vi "subTwoAntennaAlamoutiReceiver.vi"(0 "symbols in":cdb[][](array[numeric]) format="%#_6p", 5 "channel estimate":cdb[][][](array[numeric]) format="%#_6p", 11 "error in (no error)":errorcluster) -> (4 "symbols out":cdb[](array[numeric]) format="%#_6p", 15 "error out":errorcluster)   [LabVIEW 2011]
uses:
  <vilib>/Analysis/baseanly.llb/Complex A x B.vi
  <vilib>/Analysis/NI_AALBase.lvlib
panel:
  out "h matrix":cdb[][](array[numeric])
  out "branch SNRs":dbl[][](array[numeric]) format="%#_6p"
  out "combiner SNR":dbl format="%#_6p"
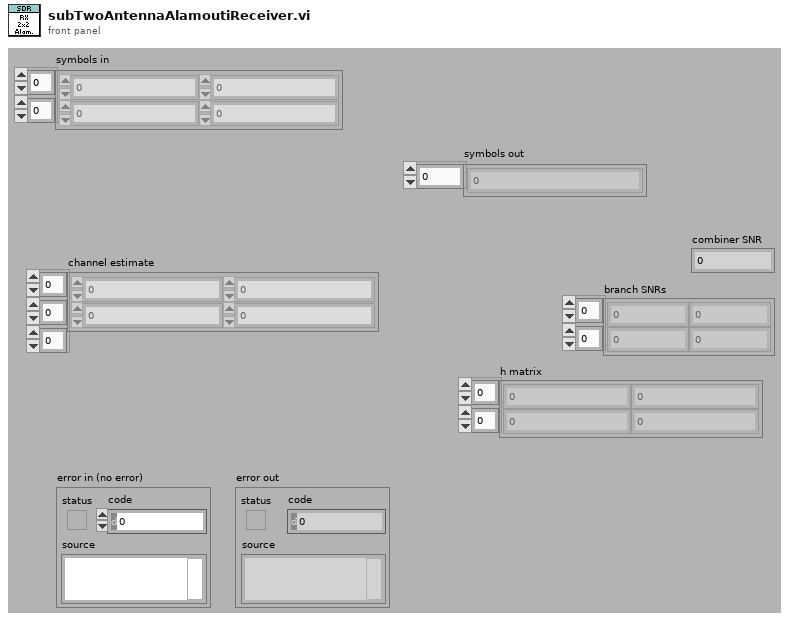
[diagram p1: front panel]
types:
  T1 = typedef "NI_Matrix.lvlib/ComplexMatrix.ctl" = cdb[][]
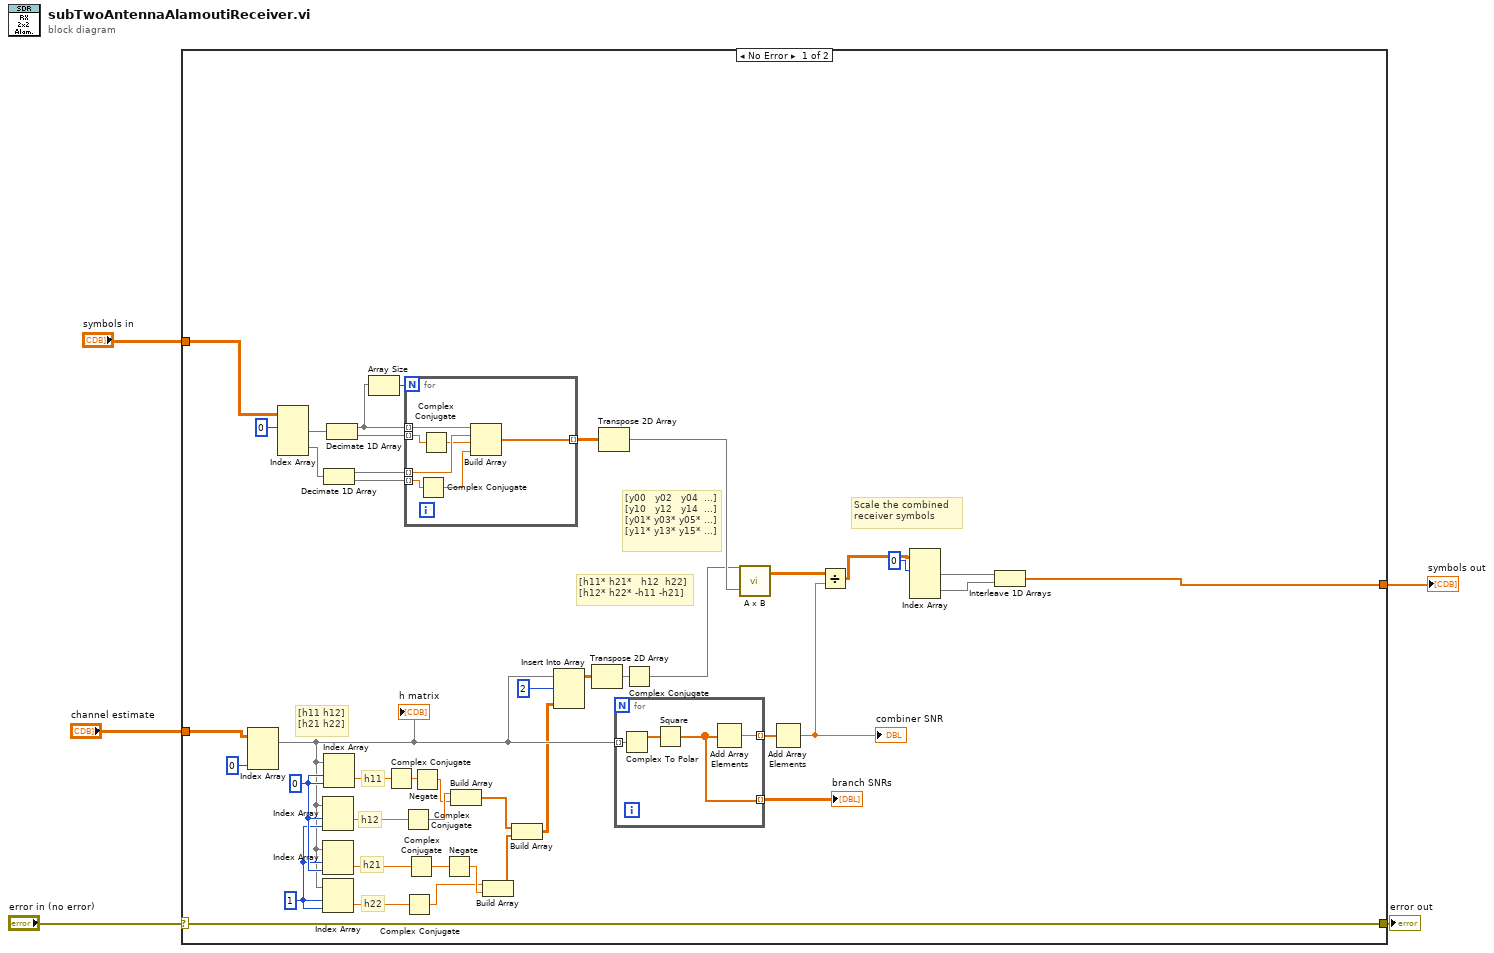
[diagram p0: block diagram]
diagram:
  n1 = case shown="No Error" "error in (no error)" {
    selector: "error in (no error)" -> [w47 w60]
    tunnel: [w47 w60] -> w4
    tunnel: "symbols in" -> [w13 _]
    tunnel: "channel estimate" -> [w12 _]
    tunnel: [w11 _] -> w1
    frame No Error {
      w42 = 1 ("index (row)")
      w43 = 0 ("index (row)")
      # "[h11* h21*   h12  h22]\n[h12* h22* -h11 -h21]"
      # "[y00   y02   y04  ...]\n[y10   y12   y14  ...]\n[y01* y03* y05* ...]\n[y11* y13* y15* ...]"
      # "h22"
      # "h21"
      # "h12"
      # "h11"
      # "[h11 h12]\n[h21 h22]"
      # "Scale the combined \nreceiver symbols"
      n2 = Index Array(array=w12, index (dim 2)=0 ("disabled index (col)")) -> (element=w31:cdb[][])  [unwired: 2 in]
      "h matrix" <- w31
      n3 = Index Array(array=w13, index (row) #1=0 ("index (row)")) -> (element #1=w16:cdb[], element #2=w15:cdb[])  [unwired: 3 in]
      n4 = Index Array(array=w31, index (row)=w43, index (col)=w42) -> (element=w39:cdb)
      n5 = Index Array(array=w31, index (row)=w42, index (col)=w43) -> (element=w40:cdb)
      n6 = Index Array(array=w31, index (row)=w42, index (col)=w42) -> (element=w41:cdb)
      n7 = Decimate 1D Array(w15) -> (w21:cdb[], w20:cdb[])
      n8 = Index Array(array=w31, index (row)=w43, index (col)=w43) -> (element=w25:cdb)
      n9 = Decimate 1D Array(w16) -> (w23:cdb[], w22:cdb[])
      n10 = Array Size(array=w23) -> (size(s)=w24:i32)
      n11 = Complex Conjugate(1:w25) -> (0:w26:cdb)
      n12 = Complex Conjugate(1:w39) -> (0:w37:cdb)
      n13 = Complex Conjugate(1:w41) -> (0:w34:cdb)
      n14 = for {
        N: w24 -> [_]
        tunnel: w23 -> [w55] mode=indexing
        tunnel: w22 -> [w54] mode=indexing
        tunnel: w21 -> [w52] mode=indexing
        tunnel: w20 -> [w53] mode=indexing
        tunnel: [w49] -> w10 mode=indexing
        n15 = Complex Conjugate(1:w53) -> (0:w50:cdb)
        n16 = Complex Conjugate(1:w54) -> (0:w51:cdb)
        n17 = Build Array(w55, w52, w51, w50) -> (w49:cdb[])
      }
      n18 = Complex Conjugate(1:w40) -> (0:w38:cdb)
      n19 = Negate(x=w26) -> (-x=w36:cdb)
      n20 = Negate(x=w38) -> (-x=w35:cdb)
      n21 = Build Array(w37, w36) -> (w32:cdb[])
      n22 = Build Array(w34, w35) -> (w33:cdb[])
      n23 = Build Array(w32, w33) -> (w29:cdb[][])
      n24 = Insert Into Array(array=w31, index (row)=2, new element=w29) -> (w27:cdb[][])  [unwired: 1 in]
      n25 = Transpose 2D Array(2D array=w27) -> (transposed array=w28:cdb[][])
      n26 = Transpose 2D Array(2D array=w10) -> (transposed array=w9:cdb[][])
      n27 = for {
        tunnel: [w58] -> w48 mode=indexing
        tunnel: [w57] -> w45 mode=indexing
        tunnel: w31 -> [w56] mode=indexing
        n28 = Complex To Polar(r * e^(i*theta)=w56) -> (r=w59:dbl[])  [unwired: 1 out]
        n29 = Square(x=w59) -> (x^2=w58:dbl[])
        n30 = Add Array Elements(numeric array=w58) -> (sum=w57:dbl)
      }
      "branch SNRs" <- w48
      n31 = Complex Conjugate(1:w28) -> (0:w8:cdb[][])
      n32 = call-poly <vilib>:"A x B.vi"("B"=w9, "A"=w8) -> ("A x B"=w7:T1)  [unwired: 1 out]
      n33 = Add Array Elements(numeric array=w45) -> (sum=w44:dbl)
      "combiner SNR" <- w44
      n34 = Divide(x=w7, y=w44) -> (x/y=w6:T1)
      n35 = Index Array(array=w6, index (row) #1=0 ("index (row)")) -> (element #1=w18:cdb[], element #2=w14:cdb[])  [unwired: 3 in]
      n36 = Interleave 1D Arrays(w18, w14) -> (w11:cdb[])
    }
    frame Error {
    }
  }
  "error out" <- w4
  "symbols out" <- w1
